vi "getADC.vi"(8 "error in (no error)":errorcluster, 10 "ILC In":refnum<class "ILC.lvclass">, 11 "ILCADC4 in":refnum<class "ILCADC4.lvclass">) -> (0 "error out":errorcluster, 1 "ADC Value":dbl[unit], 2 "ILC Out":refnum<class "ILC.lvclass">, 3 "ILCADC4 out":refnum<class "ILCADC4.lvclass">)   [LabVIEW 2015, in "ILCADC4.lvclass"]
uses:
  ILCADC4.lvclass
  <userlib>/Common/ILC/ILC/ILC.lvclass
  <userlib>/Common/ILC/ILC/ILC.lvclass/ILC.ctl
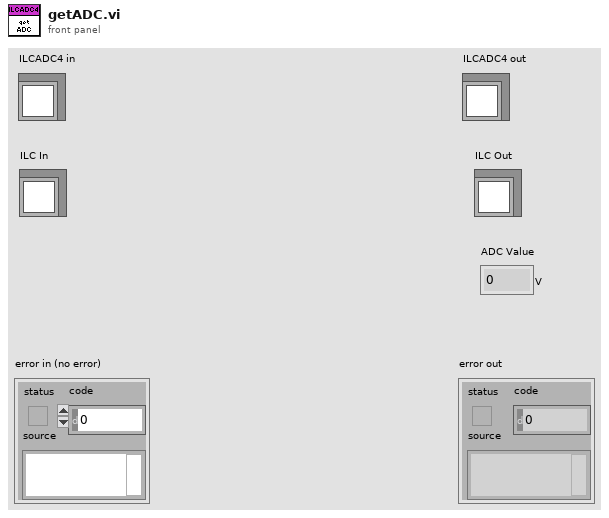
[diagram p1: front panel]
types:
  T1 = typedef "ILCCommon.lvlib/ILCTypedefs.lvlib/ADC Eng.ctl" = cluster{"Ch1":dbl[unit], "Ch2":dbl[unit], "Ch3":dbl[unit], "Ch4":dbl[unit]}
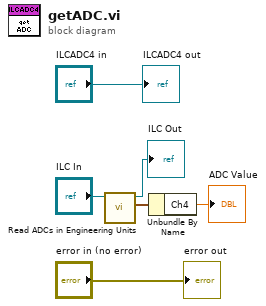
[diagram p0: block diagram]
diagram:
  n1 = call <userlib>:"Read ADCs in Engineering Units.vi"("ILC in"="ILC In") -> ("ADCs in Engineering Units"=w3:T1, "ILC out"=→"ILC Out":refnum<class "ILC.lvclass">)  [unwired: 9 in]
  n2 = Unbundle By Name(w3) -> ("Ch4"=→"ADC Value":dbl[unit])
  "error out" <- "error in (no error)"
  "ILCADC4 out" <- "ILCADC4 in"
